vi "))Channel.vi"(0 "Channel in":T1, 2 "VI Ref In":refnum<vi>, 7 "Operation":T2) -> (3 "VI Ref":refnum<vi>, 4 "Channel out":T1)   [LabVIEW 2020, in "BasicChannelWireForkable.lvlib"]
uses:
  BasicChannelWireForkable.lvlib
  Instantiate.vi
  Operation.ctl
  Element.ctl
  ))Channel.ctl
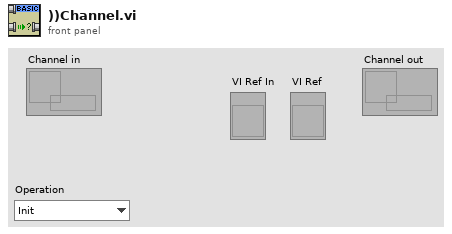
[diagram p1: front panel]
types:
  T1 = typedef "BasicChannelWireForkable.lvlib/))Channel.ctl" = refnum<queue>
  T2 = typedef "BasicChannelWireForkable.lvlib/Operation.ctl" = enum16{"Init", "Get Core", "Close"}
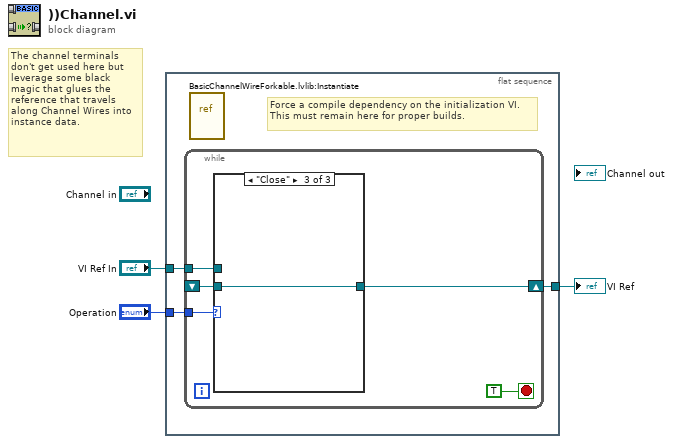
[diagram p0: block diagram]
diagram:
  # "The channel terminals don't get used here but leverage some black magic that glues the reference that travels along Channel Wires into instance data."
  n1 = flat-sequence {
    tunnel: "Operation" -> [w6]
    tunnel: "VI Ref In" -> [w5]
    tunnel: [w4] -> w1
    frame #0 {
      # "Force a compile dependency on the initialization VI. This must remain here for proper builds."
      n2 = while {
        tunnel: w6 -> [w11]
        tunnel: w5 -> [w10]
        shift-right: [w8] -> w4
        shift-left: _ -> [w7]
        stop <- TRUE stop-if-true
        n3 = case shown="\"Close\"" w11 {
          tunnel: w10 -> [w12 _ _]
          tunnel: [w12 w13 w14] -> w8
          tunnel: w7 -> [_ w13 w14]
          frame "Init" {
          }
          frame "Get Core" {
          }
          frame "Close" {
          }
        }
      }
      n4 = vi-ref "BasicChannelWireForkable.lvlib:Instantiate.vi"() -> ()  [unwired: 1 out]
    }
  }
  "VI Ref" <- w1
